vi "Untitled 3.vi"() -> ()   [LabVIEW 2026]
uses:
  <vilib>/Utility/config.llb/Read Key (String).vi
  <vilib>/Utility/config.llb/NI_LVConfig.lvlib
panel:
  out "Channels Enabled":bool[](array[boolean])
  in  "OK":bool
  in  "Sensor Name 8":string(combo)
  in  "Sensor Name 7":string(combo)
  in  "Sensor Name 6":string(combo)
  in  "Sensor Name 5":string(combo)
  in  "Sensor Name 4":string(combo)
  in  "Sensor Name 3":string(combo)
  in  "Sensor Name 2":string(combo)
  in  "Sensor Name":string(combo)
  in  "Enable/Disable  8":bool
  in  "Enable/Disable  7":bool
  in  "Enable/Disable  6":bool
  in  "Enable/Disable  5":bool
  in  "Enable/Disable  4":bool
  in  "Enable/Disable  3":bool
  in  "Enable/Disable  2":bool
  in  "Enable/Disable":bool
  in  "error in (no error)":errorcluster
  # "Channel Selection"
  # "Sensor Name"
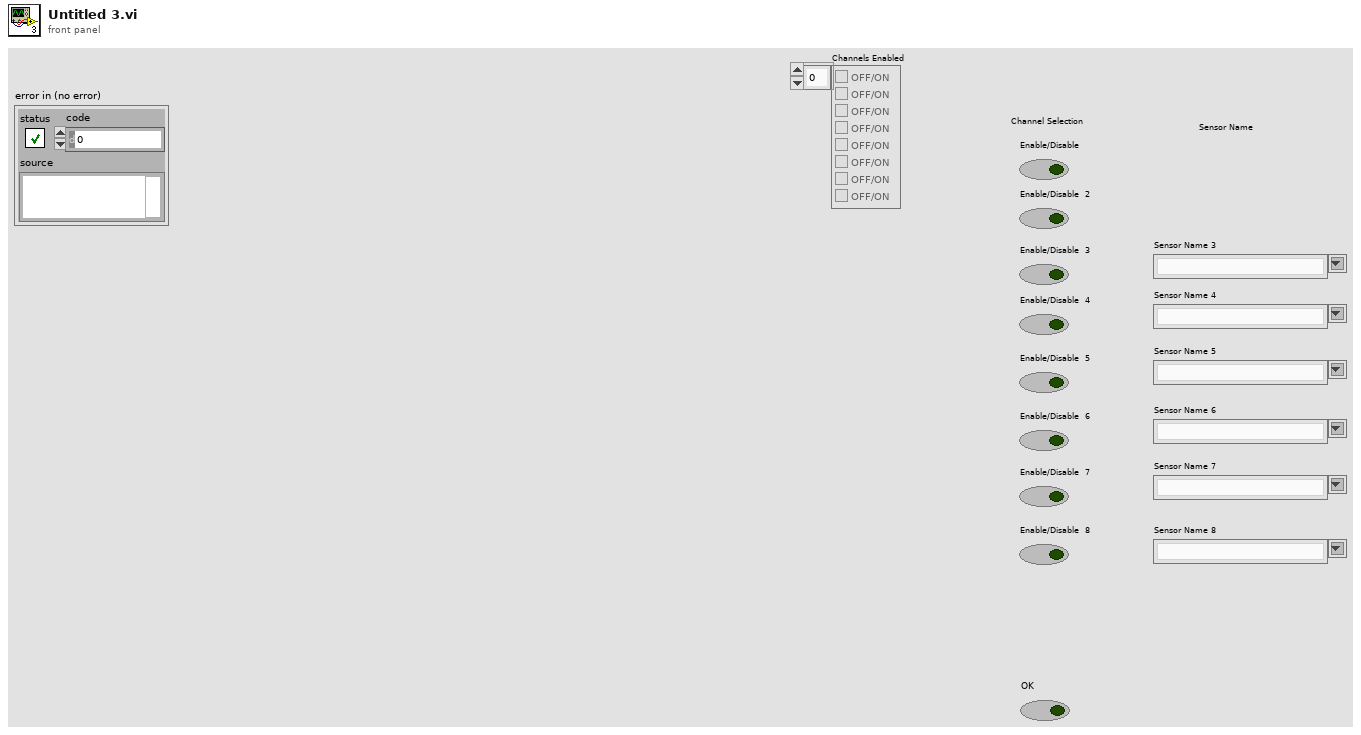
[diagram p1: front panel]
types:
  T1 = typedef "NI_LVConfig.lvlib/Config Data RefNum.ctl" = refnum<k1>
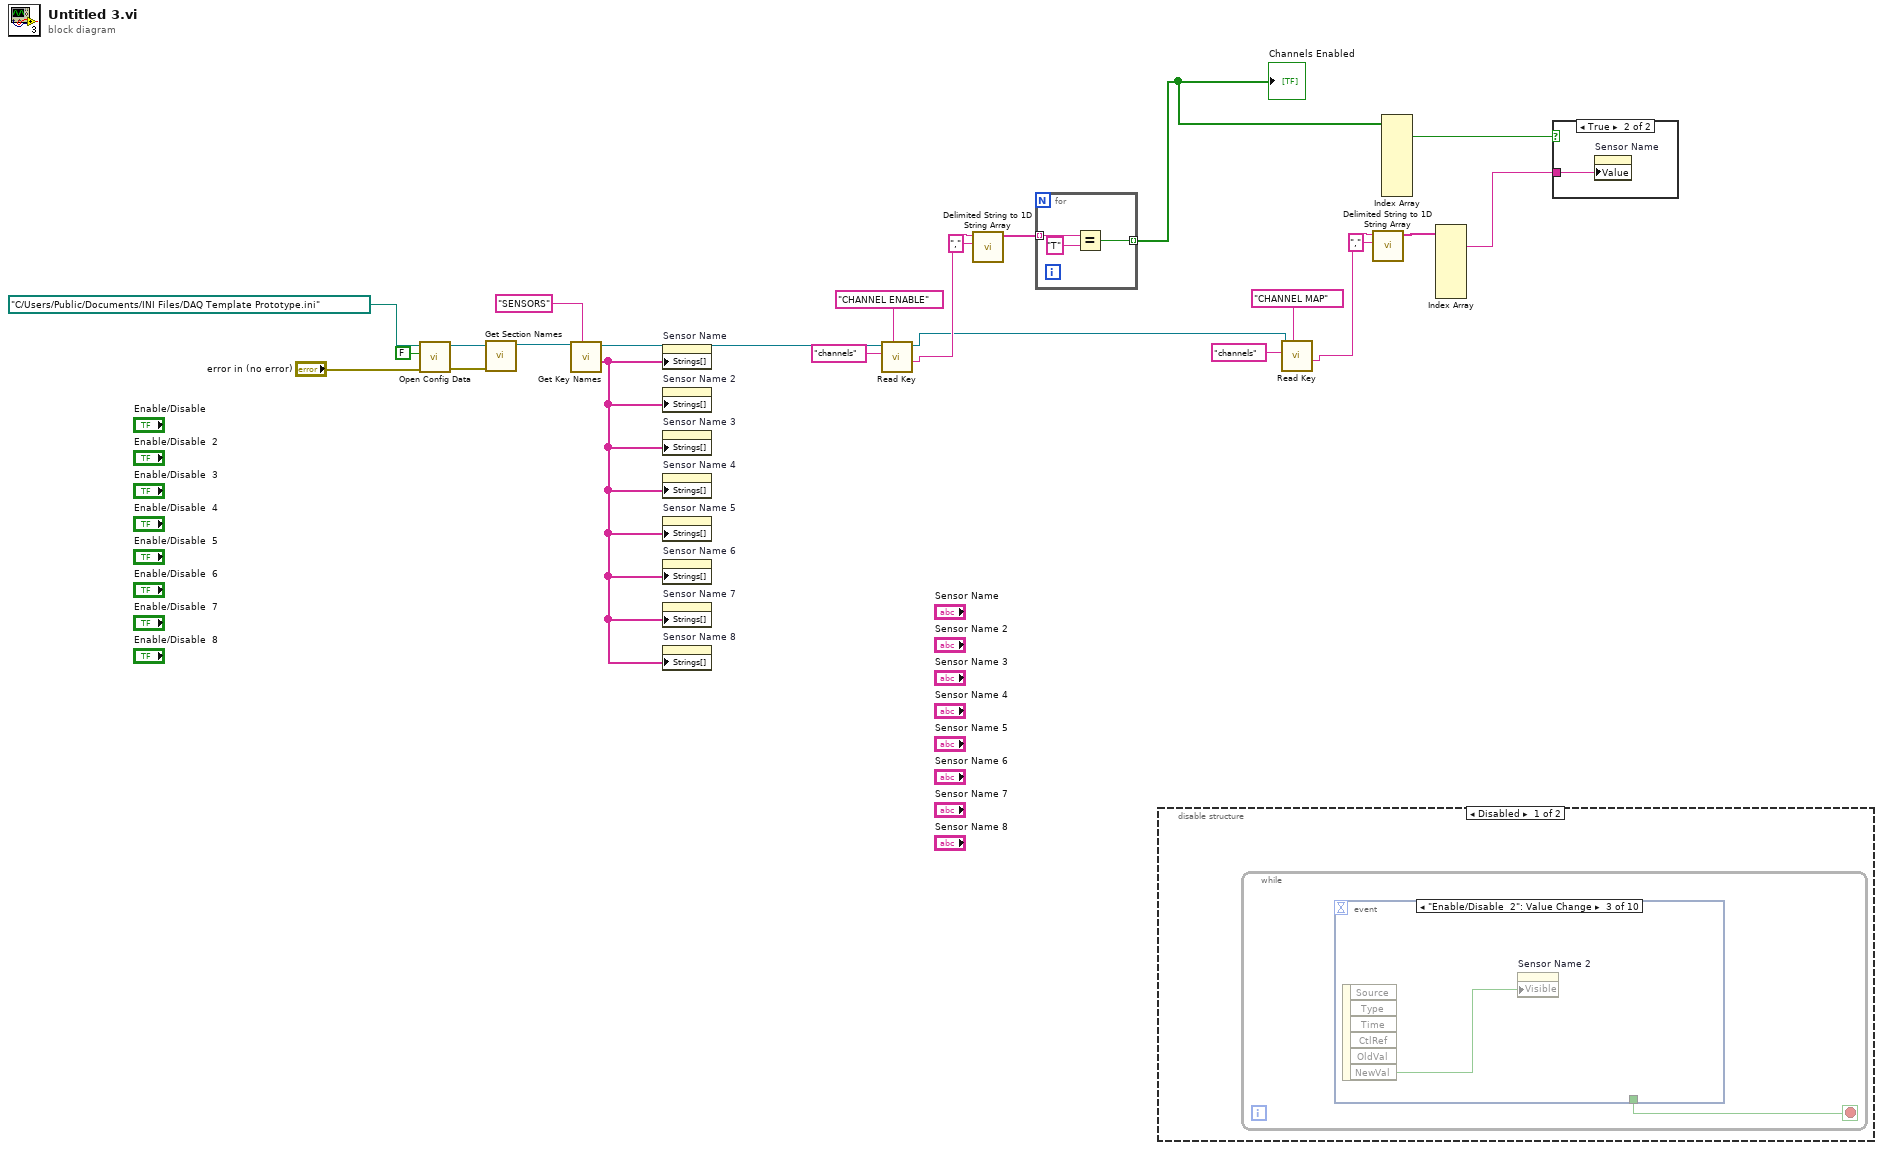
[diagram p0: block diagram]
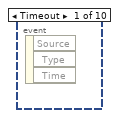
[diagram p3: hidden frame]
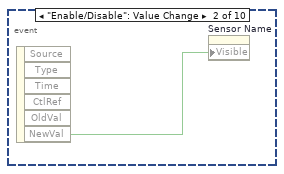
[diagram p4: hidden frame]
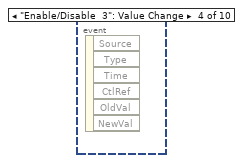
[diagram p5: hidden frame]
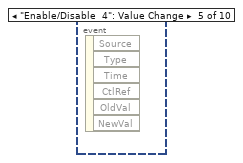
[diagram p6: hidden frame]
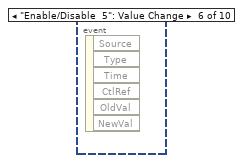
[diagram p7: hidden frame]
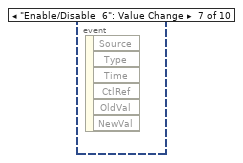
[diagram p8: hidden frame]
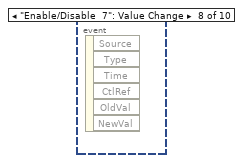
[diagram p9: hidden frame]
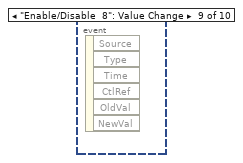
[diagram p10: hidden frame]
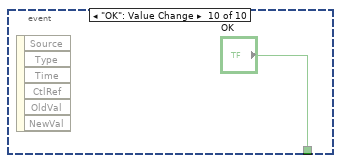
[diagram p11: hidden frame]
diagram:
  n1 = call <vilib>:"Open Config Data.vi"("error in (no error)"="error in (no error)", "create file if necessary (T)"=FALSE, "configuration file path"=path "C:/Users/Public/Documents/INI Files/DAQ Template Prototype.ini") -> ("error out"=w19:errorcluster, "refnum"=w20:T1)  [unwired: 6 in, 1 out]
  n2 = call <vilib>:"Get Section Names.vi"("error in (no error)"=w19, "refnum"=w20) -> ("refnum out"=w18:T1)  [unwired: 7 in, 2 out]
  n3 = call <vilib>:"Get Key Names.vi"("section"="SENSORS" ("y"), "refnum"=w18) -> ("key names"=w17:string[], "refnum out"=w15:T1)  [unwired: 6 in, 2 out]
  n4 = property on="Sensor Name" class="CmbBox"("Strings[]"=w17) -> ()  [unwired: 2 in, 2 out]
  n5 = property on="Sensor Name 2" class="CmbBox"("Strings[]"=w17) -> ()  [unwired: 2 in, 2 out]
  n6 = property on="Sensor Name 3" class="CmbBox"("Strings[]"=w17) -> ()  [unwired: 2 in, 2 out]
  n7 = property on="Sensor Name 4" class="CmbBox"("Strings[]"=w17) -> ()  [unwired: 2 in, 2 out]
  n8 = property on="Sensor Name 5" class="CmbBox"("Strings[]"=w17) -> ()  [unwired: 2 in, 2 out]
  n9 = property on="Sensor Name 6" class="CmbBox"("Strings[]"=w17) -> ()  [unwired: 2 in, 2 out]
  n10 = property on="Sensor Name 7" class="CmbBox"("Strings[]"=w17) -> ()  [unwired: 2 in, 2 out]
  n11 = property on="Sensor Name 8" class="CmbBox"("Strings[]"=w17) -> ()  [unwired: 2 in, 2 out]
  n12 = call-poly <vilib>:"Read Key.vi"("section"="CHANNEL ENABLE", "key"="channels", "refnum"=w15) -> ("value"=w10:string, "refnum out"=w5:T1)  [unwired: 5 in, 2 out]
  n13 = call <vilib>:"Delimited String to 1D String Array.vi"("delimiter"=",", "delimited string"=w10) -> ("string array"=w12:string[])  [unwired: 9 in]
  n14 = for {
    tunnel: w12 -> [w26] mode=indexing
    tunnel: [w24] -> w4 mode=indexing
    n15 = Equal?(x=w26, y="T") -> (x = y?=w24:bool)
  }
  "Channels Enabled" <- w4
  n16 = disable-structure shown="Disabled" {
    frame Disabled {
      n17 = while {
        stop <- w27 stop-if-true
        n18 = event shown="[2] \"Enable/Disable  2\": Value Change" {
          selector: _ -> [_ _ _ _ _ _ _ _ _ _]
          dyn-events: _ -> [_ _ _ _ _ _ _ _ _ _]
          timeout: _ -> [_ _ _ _ _ _ _ _ _ _]
          tunnel: [_ _ _ _ _ _ _ _ _ "OK"] -> w27
          event Timeout {
            n19 = event-data() -> ()  [unwired: 1 in, 3 out]
          }
          event "Enable/Disable": Value Change {
            n20 = event-data() -> ("NewVal"=w28:bool)  [unwired: 1 in, 5 out]
            n21 = property on="Sensor Name" class="CmbBox"("Visible"=w28) -> ()  [unwired: 2 in, 2 out]
          }
          event "Enable/Disable  2": Value Change {
            n22 = event-data() -> ("NewVal"=w29:bool)  [unwired: 1 in, 5 out]
            n23 = property on="Sensor Name 2" class="CmbBox"("Visible"=w29) -> ()  [unwired: 2 in, 2 out]
          }
          event "Enable/Disable  3": Value Change {
            n24 = event-data() -> ()  [unwired: 1 in, 6 out]
          }
          event "Enable/Disable  4": Value Change {
            n25 = event-data() -> ()  [unwired: 1 in, 6 out]
          }
          event "Enable/Disable  5": Value Change {
            n26 = event-data() -> ()  [unwired: 1 in, 6 out]
          }
          event "Enable/Disable  6": Value Change {
            n27 = event-data() -> ()  [unwired: 1 in, 6 out]
          }
          event "Enable/Disable  7": Value Change {
            n28 = event-data() -> ()  [unwired: 1 in, 6 out]
          }
          event "Enable/Disable  8": Value Change {
            n29 = event-data() -> ()  [unwired: 1 in, 6 out]
          }
          event "OK": Value Change {
            n30 = event-data() -> ()  [unwired: 1 in, 6 out]
          }
        }
      }
    }
    frame Enabled {
    }
  }
  n31 = call-poly <vilib>:"Read Key.vi"("section"="CHANNEL MAP", "key"="channels", "refnum"=w5) -> ("value"=w9:string)  [unwired: 5 in, 3 out]
  n32 = call <vilib>:"Delimited String to 1D String Array.vi"("delimiter"=",", "delimited string"=w9) -> ("string array"=w2:string[])  [unwired: 9 in]
  n33 = Index Array(array=w4) -> (element #1=w3:bool)  [unwired: 8 in, 7 out]
  n34 = Index Array(array=w2) -> (element #1=w1:string)  [unwired: 7 in, 6 out]
  n35 = case shown="True" w3 {
    tunnel: w1 -> [_ w31]
    frame False {
    }
    frame True {
      n36 = property on="Sensor Name" class="CmbBox"("Value"=w31) -> ()  [unwired: 2 in, 2 out]
    }
  }
